vi "Create Configuration From File.vi"(8 "error in (no error)":errorcluster, 10 "Path in":path, 11 "Device Item Ref in":T1 format="%.0x") -> (0 "error out":errorcluster, 3 "Ref out":T1 format="%.0x")   [LabVIEW 2015, in "Diagnostics Addon System Explorer.lvlib"]
uses:
  Diagnostics Addon System Explorer.lvlib
  <vilib>/NI Veristand/Custom Device API/Custom Device Item Ref.ctl
  Types/Exported Configuration.ctl
  Shared/Types/CAN Configuration.ctl
  Shared/Types/CAN Interface.ctl
  Shared/Types/Diagnostic Protocols.ctl
  Shared/Types/Transport Protocols.ctl
  Shared/Types/Security.ctl
  Types/Exported Frames Cluster.ctl
  Shared/Types/Frame Parameters.ctl
  Shared/Types/MessageType Selector.ctl
  Shared/Types/Signal Parameters.ctl
  Types/Exported DPIDs Cluster.ctl
  Types/Exported DPID Parameters.ctl
  Shared/Types/DPID Parameters.ctl
  Shared/Types/DPID Periodic Rate.ctl
  Types/Exported DTC Cluster.ctl
  Shared/Types/Exported DTC Control Cluster.ctl
  Types/Exported 986x Support.ctl
  Types/Exported Command Cluster.ctl
  Types/Exported Status Cluster.ctl
  Shared/Types/Exported IO Control Cluster.ctl
  Shared/Types/IO Control Parameters.ctl
  Shared/Types/Command Response Signals.ctl
  Shared/Types/Exported Routines Cluster.ctl
  Shared/Types/Routine Paramaters.ctl
  <vilib>/NI/GXML/_subVIs/GXML SearchParser/Search Parser.vi
  <vilib>/NI/GXML/GXML.lvlib
  Shared/Diagnostics Addon Shared.lvlib
  <vilib>/NI Veristand/Custom Device API/Custom Device API.lvlib
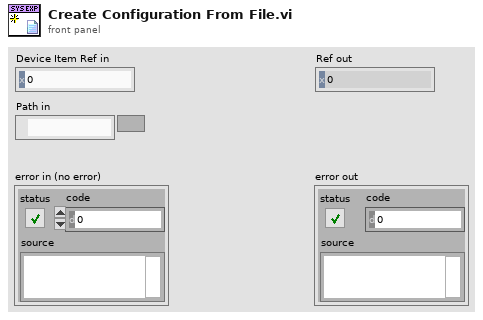
[diagram p1: front panel]
types:
  T1 = typedef "Custom Device API.lvlib/Custom Device Item Ref.ctl" = u64
  T2 = cluster{"Name":string, "Description":string, "Diagnostics Basic Configuraiton":cluster{"Database File":path, "CAN Interface":enum16{"CAN0", "CAN1", "CAN2", "CAN3", "CAN4", "CAN5", "CAN6", "CAN7", "CAN8", "CAN9", "CAN10", "CAN11", "CAN12", "CAN13", "CAN14", "CAN15", "CAN16", "CAN17", "CAN18", "CAN19", "CAN20", "CAN21", "CAN22", "CAN23", "CAN24", "CAN25", "CAN26", "CAN27", "CAN28", "CAN29", "CAN30", "CAN31", "CAN32", "CAN33", "CAN34", "CAN35", "CAN36", "CAN37", "CAN38", "CAN39", "CAN40", "CAN41", "CAN42", "CAN43", "CAN44", "CAN45", "CAN46", "CAN47", "CAN48", "CAN49", "CAN50", "CAN51", "CAN52", "CAN53", "CAN54", "CAN55", "CAN56", "CAN57", "CAN58", "CAN59", "CAN60", "CAN61", "CAN62", "CAN63", "CAN 256 (Virtual)", "CAN 257 (Virtual)"}, "Baud Rate":u32, "Diagnostic Protocol":enum16{"GMLAN", "KWP-2000", "UDS"}, "Transport Protocol":enum16{"ISO TP - Normal Mode", "ISO TP - Mixed Mode", "VW TP 2.0", "Diagnostics on IP"}, "Transmit ID":u32, "Receive ID":u32, "Transmit Extension":u8, "Receive Extension":u8, "Receive UUDT ID":u32, "Enable Stream":bool, "VW TP Channel ID":u32}, "DIDs":cluster{"Description":string, "DIDPID Array":cluster{"Name":string, "Description":string, "ID":u16, "Signals":cluster{"Name":string, "Start Bit":u8, "Length":u8, "Scaling Factor":dbl, "Scaling Offset":dbl, "Minimum":dbl, "Maximum":dbl, "Data Type":u32, "Byte Order":u32, "Default Value":dbl, "Units":string, "Description":string}[]}[]}, "Input PIDs":cluster{"Description":string, "DIDPID Array":cluster{"Name":string, "Description":string, "ID":u16, "Signals":cluster{"Name":string, "Start Bit":u8, "Length":u8, "Scaling Factor":dbl, "Scaling Offset":dbl, "Minimum":dbl, "Maximum":dbl, "Data Type":u32, "Byte Order":u32, "Default Value":dbl, "Units":string, "Description":string}[]}[]}, "Output PIDs":cluster{"Description":string, "DIDPID Array":cluster{"Name":string, "Description":string, "ID":u16, "Signals":cluster{"Name":string, "Start Bit":u8, "Length":u8, "Scaling Factor":dbl, "Scaling Offset":dbl, "Minimum":dbl, "Maximum":dbl, "Data Type":u32, "Byte Order":u32, "Default Value":dbl, "Units":string, "Description":string}[]}[]}, "DPIDs":cluster{"Description":string, "DPIDs":cluster{"Name":string, "Description":string, "DPID":cluster{"DPID ID":u8, "Speed":enum16{"Slow", "Medium", "Fast"}, "PIDs":u16[]}}[]}, "DTC":cluster{"Description":string, "DTC descriptor":cluster{"DTC Byte Length":i32, "Status Byte Length":i32, "Add Data Byte Length":i32, "Byte Order":enum16{"Motorola", "Intel"}}}, "NI 986x Support":cluster{"Enable 986x":bool, "RIO Device":u16, "Bitfile":path}, "Commands":cluster{"Description":string}, "Status":cluster{"Description":string}}
  T3 = typedef "Diagnostics Addon System Explorer.lvlib/Exported Configuration.ctl" = cluster{"Name":string, "Description":string, "Diagnostics Basic Configuraiton":T4, "DIDs":T9, "Input PIDs":T9, "Output PIDs":T9, "DPIDs":T13, "DTC":T17, "NI 986x Support":T19, "Commands":T20, "Status":T21, "IO Controls":T22, "Routines":T25, "Output Memory":T9, "Input Memory":T9}
  T4 = typedef "Diagnostics Addon Shared.lvlib/CAN Configuration.ctl" = cluster{"Database File":path, "CAN Interface":T5, "Baud Rate":u32, "Diagnostic Protocol":T6, "Transport Protocol":T7, "Transmit ID":u32, "Receive ID":u32, "Transmit Extension":u8, "Receive Extension":u8, "Receive UUDT ID":u32, "Enable Stream":bool, "VW TP Channel ID":u32, "Security":T8, "Fill Frame":bool, "Fill Byte":u8, "Termination":bool}
  T5 = typedef "Diagnostics Addon Shared.lvlib/CAN Interface.ctl" = enum16{"CAN0", "CAN1", "CAN2", "CAN3", "CAN4", "CAN5", "CAN6", "CAN7", "CAN8", "CAN9", "CAN10", "CAN11", "CAN12", "CAN13", "CAN14", "CAN15", "CAN16", "CAN17", "CAN18", "CAN19", "CAN20", "CAN21", "CAN22", "CAN23", "CAN24", "CAN25", "CAN26", "CAN27", "CAN28", "CAN29", "CAN30", "CAN31", "CAN32", "CAN33", "CAN34", "CAN35", "CAN36", "CAN37", "CAN38", "CAN39", "CAN40", "CAN41", "CAN42", "CAN43", "CAN44", "CAN45", "CAN46", "CAN47", "CAN48", "CAN49", "CAN50", "CAN51", "CAN52", "CAN53", "CAN54", "CAN55", "CAN56", "CAN57", "CAN58", "CAN59", "CAN60", "CAN61", "CAN62", "CAN63", "CAN 256 (Virtual)", "CAN 257 (Virtual)"}
  T6 = typedef "Diagnostics Addon Shared.lvlib/Diagnostic Protocols.ctl" = enum16{"GMLAN", "KWP-2000", "UDS"}
  T7 = typedef "Diagnostics Addon Shared.lvlib/Transport Protocols.ctl" = enum16{"ISO TP - Normal Mode", "ISO TP - Mixed Mode", "VW TP 2.0", "Diagnostics on IP"}
  T8 = typedef "Diagnostics Addon Shared.lvlib/Security.ctl" = cluster{"Source DLL Path":path, "Security Level":u8, "Target DLL Path":path}
  T9 = typedef "Diagnostics Addon System Explorer.lvlib/Exported Frames Cluster.ctl" = cluster{"Description":string, "Frames":T10[]}
  T10 = typedef "Diagnostics Addon Shared.lvlib/Frame Parameters.ctl" = cluster{"Name":string, "Description":string, "ID":u32, "Type":T11, "Signals":T12[]}
  T11 = typedef "Diagnostics Addon Shared.lvlib/MessageType Selector.ctl" = enum16{"DID", "PID", "CPID", "Write Memory", "Read Memory", "DTC Control", "IO Cmd", "IO Resp", "Routine Start Cmd", "Routine Start Resp", "Routine Status Cmd", "Routine Status Resp", "Routine Stop Cmd", "Routine Stop Resp"}
  T12 = typedef "Diagnostics Addon Shared.lvlib/Signal Parameters.ctl" = cluster{"Start Bit":u8, "Length":u8, "Scaling Factor":dbl, "Scaling Offset":dbl, "Minimum":dbl, "Maximum":dbl, "Data Type":u32, "Byte Order":u32, "Default Value":dbl, "Name":string, "Units":string, "Description":string}
  T13 = typedef "Diagnostics Addon System Explorer.lvlib/Exported DPIDs Cluster.ctl" = cluster{"Description":string, "DPIDs":T14[]}
  T14 = typedef "Diagnostics Addon System Explorer.lvlib/Exported DPID Parameters.ctl" = cluster{"Name":string, "Description":string, "DPID":T15}
  T15 = typedef "Diagnostics Addon Shared.lvlib/DPID Parameters.ctl" = cluster{"DPID ID":u8, "Speed":T16, "PIDs":u16[]}
  T16 = typedef "Diagnostics Addon Shared.lvlib/DPID Periodic Rate.ctl" = enum16{"Slow", "Medium", "Fast"}
  T17 = typedef "Diagnostics Addon System Explorer.lvlib/Exported DTC Cluster.ctl" = cluster{"Description":string, "DTC descriptor":cluster{"DTC Byte Length":i32, "Status Byte Length":i32, "Add Data Byte Length":i32, "Byte Order":enum16{"Motorola", "Intel"}}, "DTCControl":T18}
  T18 = typedef "Diagnostics Addon Shared.lvlib/Exported DTC Control Cluster.ctl" = cluster{"Description":string, "Signals":T12[]}
  T19 = typedef "Diagnostics Addon System Explorer.lvlib/Exported 986x Support.ctl" = cluster{"Enable 986x":bool, "RIO Device":u16, "Bitfile":path}
  T20 = typedef "Diagnostics Addon System Explorer.lvlib/Exported Command Cluster.ctl" = cluster{"Description":string}
  T21 = typedef "Diagnostics Addon System Explorer.lvlib/Exported Status Cluster.ctl" = cluster{"Description":string}
  T22 = typedef "Diagnostics Addon Shared.lvlib/Exported IO Control Cluster.ctl" = cluster{"Description":string, "IO Control Array":T23[]}
  T23 = typedef "Diagnostics Addon Shared.lvlib/IO Control Parameters.ctl" = cluster{"Name":string, "Description":string, "ID":u16, "Signals":T24}
  T24 = typedef "Diagnostics Addon Shared.lvlib/Command Response Signals.ctl" = cluster{"Cmd":T12[], "Response":T12[]}
  T25 = typedef "Diagnostics Addon Shared.lvlib/Exported Routines Cluster.ctl" = cluster{"Description":string, "Routine Array":T26[]}
  T26 = typedef "Diagnostics Addon Shared.lvlib/Routine Paramaters.ctl" = cluster{"Name":string, "Description":string, "ID":u16, "Start Parameters":T24, "Request Parameters":T24, "Stop Parameters":T24}
  T27 = cluster{"Description":string, "DPIDs":cluster{"Name":string, "Description":string, "DPID":cluster{"DPID ID":u8, "Speed":enum16{"Slow", "Medium", "Fast"}, "PIDs":u16[]}}[]}
  T28 = cluster{"DTC Byte Length":i32, "Status Byte Length":i32, "Add Data Byte Length":i32, "Byte Order":enum16{"Motorola", "Intel"}}
  T29 = cluster{"Enable 986x":bool, "RIO Device":u16, "Bitfile":path}
  T30 = enum16{"CAN0", "CAN1", "CAN2", "CAN3", "CAN4", "CAN5", "CAN6", "CAN7", "CAN8", "CAN9", "CAN10", "CAN11", "CAN12", "CAN13", "CAN14", "CAN15", "CAN16", "CAN17", "CAN18", "CAN19", "CAN20", "CAN21", "CAN22", "CAN23", "CAN24", "CAN25", "CAN26", "CAN27", "CAN28", "CAN29", "CAN30", "CAN31", "CAN32", "CAN33", "CAN34", "CAN35", "CAN36", "CAN37", "CAN38", "CAN39", "CAN40", "CAN41", "CAN42", "CAN43", "CAN44", "CAN45", "CAN46", "CAN47", "CAN48", "CAN49", "CAN50", "CAN51", "CAN52", "CAN53", "CAN54", "CAN55", "CAN56", "CAN57", "CAN58", "CAN59", "CAN60", "CAN61", "CAN62", "CAN63", "CAN 256 (Virtual)", "CAN 257 (Virtual)"}
  T31 = enum16{"ISO TP - Normal Mode", "ISO TP - Mixed Mode", "VW TP 2.0", "Diagnostics on IP"}
  T32 = cluster{"Name":string, "Description":string, "ID":u16, "Signals":cluster{"Name":string, "Start Bit":u8, "Length":u8, "Scaling Factor":dbl, "Scaling Offset":dbl, "Minimum":dbl, "Maximum":dbl, "Data Type":u32, "Byte Order":u32, "Default Value":dbl, "Units":string, "Description":string}[]}[]
  T33 = cluster{"Name":string, "Description":string, "Diagnostics Basic Configuraiton":cluster{"Database File":path, "CAN Interface":enum16{"CAN0", "CAN1", "CAN2", "CAN3", "CAN4", "CAN5", "CAN6", "CAN7", "CAN8", "CAN9", "CAN10", "CAN11", "CAN12", "CAN13", "CAN14", "CAN15", "CAN16", "CAN17", "CAN18", "CAN19", "CAN20", "CAN21", "CAN22", "CAN23", "CAN24", "CAN25", "CAN26", "CAN27", "CAN28", "CAN29", "CAN30", "CAN31", "CAN32", "CAN33", "CAN34", "CAN35", "CAN36", "CAN37", "CAN38", "CAN39", "CAN40", "CAN41", "CAN42", "CAN43", "CAN44", "CAN45", "CAN46", "CAN47", "CAN48", "CAN49", "CAN50", "CAN51", "CAN52", "CAN53", "CAN54", "CAN55", "CAN56", "CAN57", "CAN58", "CAN59", "CAN60", "CAN61", "CAN62", "CAN63", "CAN 256 (Virtual)", "CAN 257 (Virtual)"}, "Baud Rate":u32, "Diagnostic Protocol":enum16{"GMLAN", "KWP-2000", "UDS"}, "Transport Protocol":enum16{"ISO TP - Normal Mode", "ISO TP - Mixed Mode", "VW TP 2.0", "Diagnostics on IP"}, "Transmit ID":u32, "Receive ID":u32, "Transmit Extension":u8, "Receive Extension":u8, "Receive UUDT ID":u32, "Enable Stream":bool, "VW TP Channel ID":u32}, "DIDs":cluster{"Description":string, "DIDPID Array":cluster{"Name":string, "Description":string, "ID":u16, "Signals":cluster{"Start Bit":u8, "Length":u8, "Scaling Factor":dbl, "Scaling Offset":dbl, "Minimum":dbl, "Maximum":dbl, "Data Type":u32, "Byte Order":u32, "Default Value":dbl, "Name":string, "Units":string, "Description":string}[]}[]}, "Input PIDs":cluster{"Description":string, "DIDPID Array":cluster{"Name":string, "Description":string, "ID":u16, "Signals":cluster{"Start Bit":u8, "Length":u8, "Scaling Factor":dbl, "Scaling Offset":dbl, "Minimum":dbl, "Maximum":dbl, "Data Type":u32, "Byte Order":u32, "Default Value":dbl, "Name":string, "Units":string, "Description":string}[]}[]}, "Output PIDs":cluster{"Description":string, "DIDPID Array":cluster{"Name":string, "Description":string, "ID":u16, "Signals":cluster{"Start Bit":u8, "Length":u8, "Scaling Factor":dbl, "Scaling Offset":dbl, "Minimum":dbl, "Maximum":dbl, "Data Type":u32, "Byte Order":u32, "Default Value":dbl, "Name":string, "Units":string, "Description":string}[]}[]}, "DPIDs":cluster{"Description":string, "DPIDs":cluster{"Name":string, "Description":string, "DPID":cluster{"DPID ID":u8, "Speed":enum16{"Slow", "Medium", "Fast"}, "PIDs":u16[]}}[]}, "DTC":cluster{"Description":string, "DTC descriptor":cluster{"DTC Byte Length":i32, "Status Byte Length":i32, "Add Data Byte Length":i32, "Byte Order":enum16{"Motorola", "Intel"}}}, "NI 986x Support":cluster{"Enable 986x":bool, "RIO Device":u16, "Bitfile":path}, "Commands":cluster{"Description":string}, "Status":cluster{"Description":string}}
  T34 = cluster{"Name":string, "Description":string, "ID":u16, "Signals":cluster{"Start Bit":u8, "Length":u8, "Scaling Factor":dbl, "Scaling Offset":dbl, "Minimum":dbl, "Maximum":dbl, "Data Type":u32, "Byte Order":u32, "Default Value":dbl, "Name":string, "Units":string, "Description":string}[]}[]
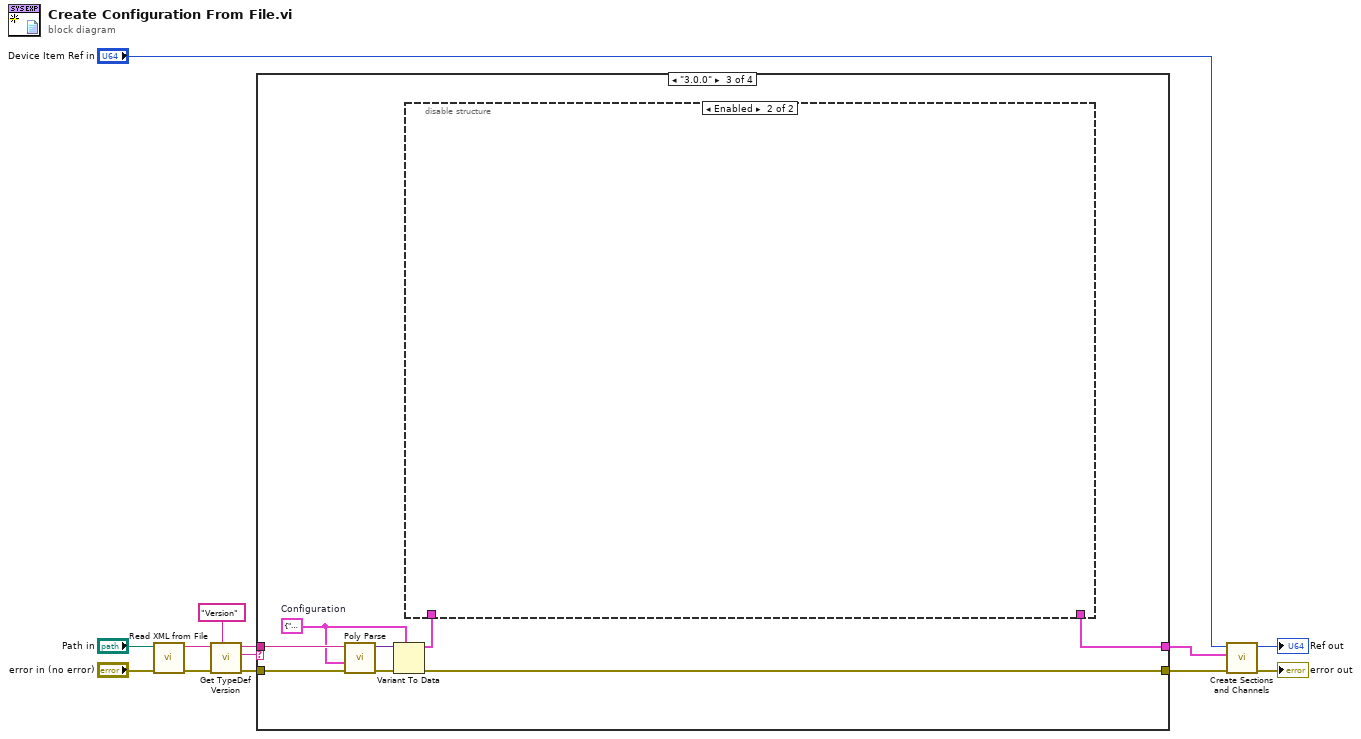
[diagram p0: block diagram]
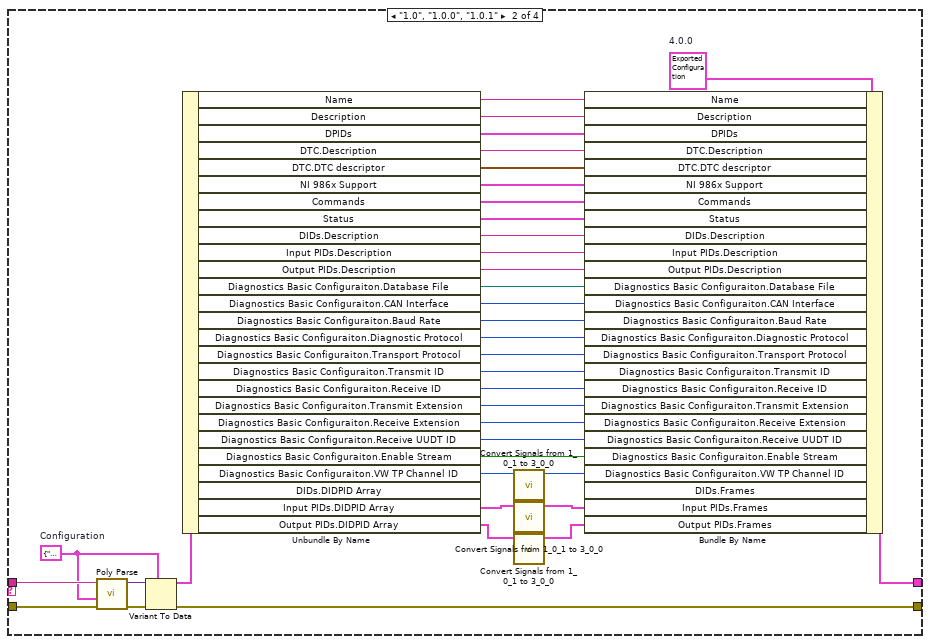
[diagram p3: hidden frame]
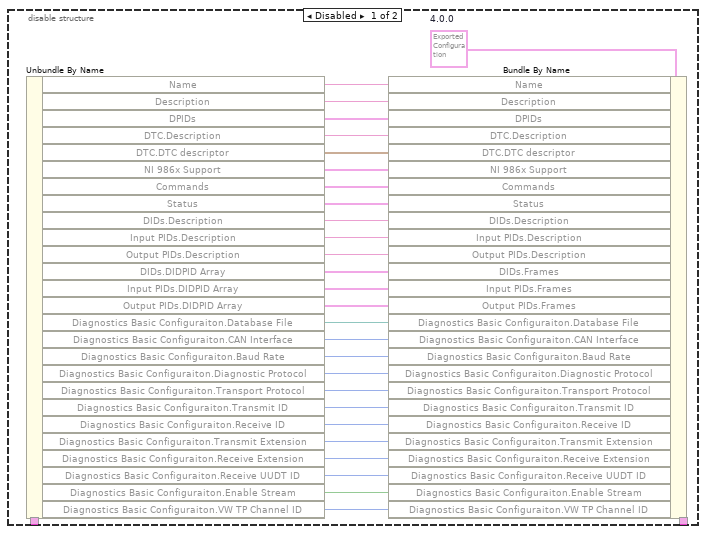
[diagram p4: hidden frame]
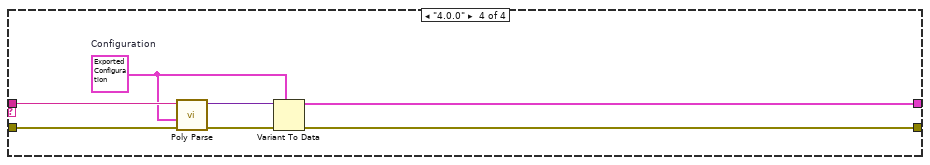
[diagram p5: hidden frame]
diagram:
  n1 = call <vilib>:"Read XML from File.vi"("error in"="error in (no error)", "XML File Path"="Path in") -> ("error out"=w13:errorcluster, "XML String Out"=w12:string)  [unwired: 8 in]
  n2 = call <vilib>:"Get TypeDef Version.vi"("Version Tag Name"="Version", "error in"=w13, "XML String In"=w12) -> ("error out"=w9:errorcluster, "Version String"=w8:string, "XML String Out"=w10:string)  [unwired: 6 in]
  n3 = case shown="\"3.0.0\"" w8 {
    tunnel: w10 -> [_ w52 w60 w96]
    tunnel: w9 -> [w14 w51 w59 w95]
    tunnel: [_ w35 w54 w92] -> w1
    tunnel: [w14 w48 w56 w90] -> w5
    frame Default {
    }
    frame "1.0", "1.0.0", "1.0.1" {
      w34 = T2 {"Name"="", "Description"="", "Diagnostics Basic Configuraiton"={"Database File"=path "", "CAN Interface"=enum."CAN0", "Baud Rate"=0, "Diagnostic Protocol"=enum."GMLAN", "Transport Protocol"=enum."ISO TP - Normal Mode", "Transmit ID"=0, "Receive ID"=0, "Transmit Extension"=0, "Receive Extension"=0, "Receive UUDT ID"=0, "Enable Stream"=FALSE, "VW TP Channel ID"=0}, "DIDs"={"Description"="", "DIDPID Array"=[]}, "Input PIDs"={"Description"="", "DIDPID Array"=[]}, "Output PIDs"={"Description"="", "DIDPID Array"=[]}, "DPIDs"={"Description"="", "DPIDs"=[]}, "DTC"={"Description"="", "DTC descriptor"={"DTC Byte Length"=0, "Status Byte Length"=0, "Add Data Byte Length"=0, "Byte Order"=enum."Motorola"}}, "NI 986x Support"={"Enable 986x"=FALSE, "RIO Device"=0, "Bitfile"=path ""}, "Commands"={"Description"=""}, "Status"={"Description"=""}}  # Configuration
      w46 = T3 {"Name"="", "Description"="", "Diagnostics Basic Configuraiton"={"Database File"=path "", "CAN Interface"=enum."CAN0", "Baud Rate"=0, "Diagnostic Protocol"=enum."GMLAN", "Transport Protocol"=enum."ISO TP - Normal Mode", "Transmit ID"=0, "Receive ID"=0, "Transmit Extension"=0, "Receive Extension"=0, "Receive UUDT ID"=0, "Enable Stream"=FALSE, "VW TP Channel ID"=0, "Security"={"Source DLL Path"=path "", "Security Level"=1, "Target DLL Path"=path ""}, "Fill Frame"=FALSE, "Fill Byte"=255, "Termination"=FALSE}, "DIDs"={"Description"="", "Frames"=[]}, "Input PIDs"={"Description"="", "Frames"=[]}, "Output PIDs"={"Description"="", "Frames"=[]}, "DPIDs"={"Description"="", "DPIDs"=[]}, "DTC"={"Description"="", "DTC descriptor"={"DTC Byte Length"=0, "Status Byte Length"=0, "Add Data Byte Length"=0, "Byte Order"=enum."Motorola"}, "DTCControl"={"Description"="", "Signals"=[]}}, "NI 986x Support"={"Enable 986x"=FALSE, "RIO Device"=0, "Bitfile"=path ""}, "Commands"={"Description"=""}, "Status"={"Description"=""}, "IO Controls"={"Description"="", "IO Control Array"=[]}, "Routines"={"Description"="", "Routine Array"=[]}, "Output Memory"={"Description"="", "Frames"=[]}, "Input Memory"={"Description"="", "Frames"=[]}}  # 4.0.0
      n4 = call-poly <vilib>:"Poly Parse.vi"("error in"=w51, "TypeDesc"=w34, "XML String In"=w52) -> ("error out"=w50:errorcluster, "Parsed Data"=w49:variant)  [unwired: 7 in]
      n5 = Variant To Data(error in=w50, type=w34, Variant=w49) -> (data=w47:T2, error out=w48:errorcluster)
      n6 = Unbundle By Name(w47) -> ("Name"=w45:string, "Description"=w44:string, "DPIDs"=w43:T27, "DTC.Description"=w39:string, "DTC.DTC descriptor"=w15:T28, "NI 986x Support"=w40:T29, "Commands"=w41:cluster{"Description":string}, "Status"=w42:cluster{"Description":string}, "DIDs.Description"=w38:string, "Input PIDs.Description"=w37:string, "Output PIDs.Description"=w36:string, "Diagnostics Basic Configuraiton.Database File"=w22:path, "Diagnostics Basic Configuraiton.CAN Interface"=w23:T30, "Diagnostics Basic Configuraiton.Baud Rate"=w24:u32, "Diagnostics Basic Configuraiton.Diagnostic Protocol"=w25:enum16{"GMLAN", "KWP-2000", "UDS"}, "Diagnostics Basic Configuraiton.Transport Protocol"=w26:T31, "Diagnostics Basic Configuraiton.Transmit ID"=w27:u32, "Diagnostics Basic Configuraiton.Receive ID"=w28:u32, "Diagnostics Basic Configuraiton.Transmit Extension"=w29:u8, "Diagnostics Basic Configuraiton.Receive Extension"=w30:u8, "Diagnostics Basic Configuraiton.Receive UUDT ID"=w31:u32, "Diagnostics Basic Configuraiton.Enable Stream"=w32:bool, "Diagnostics Basic Configuraiton.VW TP Channel ID"=w33:u32, "DIDs.DIDPID Array"=w21:T32, "Input PIDs.DIDPID Array"=w20:T32, "Output PIDs.DIDPID Array"=w19:T32)
      n7 = call "Convert Signals from 1_0_1 to 3_0_0.vi"("Signals"=w21) -> ("Signals"=w18:T10[])  [unwired: 10 in]
      n8 = call "Convert Signals from 1_0_1 to 3_0_0.vi"("Signals"=w20) -> ("Signals"=w17:T10[])  [unwired: 10 in]
      n9 = call "Convert Signals from 1_0_1 to 3_0_0.vi"("Signals"=w19) -> ("Signals"=w16:T10[])  [unwired: 10 in]
      n10 = Bundle By Name(cluster=w46, "Name"=w45, "Description"=w44, "DPIDs"=w43, "DTC.Description"=w39, "DTC.DTC descriptor"=w15, "NI 986x Support"=w40, "Commands"=w41, "Status"=w42, "DIDs.Description"=w38, "Input PIDs.Description"=w37, "Output PIDs.Description"=w36, "Diagnostics Basic Configuraiton.Database File"=w22, "Diagnostics Basic Configuraiton.CAN Interface"=w23, "Diagnostics Basic Configuraiton.Baud Rate"=w24, "Diagnostics Basic Configuraiton.Diagnostic Protocol"=w25, "Diagnostics Basic Configuraiton.Transport Protocol"=w26, "Diagnostics Basic Configuraiton.Transmit ID"=w27, "Diagnostics Basic Configuraiton.Receive ID"=w28, "Diagnostics Basic Configuraiton.Transmit Extension"=w29, "Diagnostics Basic Configuraiton.Receive Extension"=w30, "Diagnostics Basic Configuraiton.Receive UUDT ID"=w31, "Diagnostics Basic Configuraiton.Enable Stream"=w32, "Diagnostics Basic Configuraiton.VW TP Channel ID"=w33, "DIDs.Frames"=w18, "Input PIDs.Frames"=w17, "Output PIDs.Frames"=w16) -> (w35:T3)
    }
    frame "3.0.0" {
      w53 = T33 {"Name"="", "Description"="", "Diagnostics Basic Configuraiton"={"Database File"=path "", "CAN Interface"=enum."CAN0", "Baud Rate"=0, "Diagnostic Protocol"=enum."GMLAN", "Transport Protocol"=enum."ISO TP - Normal Mode", "Transmit ID"=0, "Receive ID"=0, "Transmit Extension"=0, "Receive Extension"=0, "Receive UUDT ID"=0, "Enable Stream"=FALSE, "VW TP Channel ID"=0}, "DIDs"={"Description"="", "DIDPID Array"=[]}, "Input PIDs"={"Description"="", "DIDPID Array"=[]}, "Output PIDs"={"Description"="", "DIDPID Array"=[]}, "DPIDs"={"Description"="", "DPIDs"=[]}, "DTC"={"Description"="", "DTC descriptor"={"DTC Byte Length"=0, "Status Byte Length"=0, "Add Data Byte Length"=0, "Byte Order"=enum."Motorola"}}, "NI 986x Support"={"Enable 986x"=FALSE, "RIO Device"=0, "Bitfile"=path ""}, "Commands"={"Description"=""}, "Status"={"Description"=""}}  # Configuration
      n11 = call-poly <vilib>:"Poly Parse.vi"("error in"=w59, "TypeDesc"=w53, "XML String In"=w60) -> ("error out"=w58:errorcluster, "Parsed Data"=w57:variant)  [unwired: 7 in]
      n12 = Variant To Data(error in=w58, type=w53, Variant=w57) -> (data=w55:T33, error out=w56:errorcluster)
      n13 = disable-structure shown="Enabled" {
        disable-tunnel: w55 -> [w89 _]
        disable-tunnel: [w77 _] -> w54
        frame Disabled {
          w88 = T3 {"Name"="", "Description"="", "Diagnostics Basic Configuraiton"={"Database File"=path "", "CAN Interface"=enum."CAN0", "Baud Rate"=0, "Diagnostic Protocol"=enum."GMLAN", "Transport Protocol"=enum."ISO TP - Normal Mode", "Transmit ID"=0, "Receive ID"=0, "Transmit Extension"=0, "Receive Extension"=0, "Receive UUDT ID"=0, "Enable Stream"=FALSE, "VW TP Channel ID"=0, "Security"={"Source DLL Path"=path "", "Security Level"=1, "Target DLL Path"=path ""}, "Fill Frame"=FALSE, "Fill Byte"=255, "Termination"=FALSE}, "DIDs"={"Description"="", "Frames"=[]}, "Input PIDs"={"Description"="", "Frames"=[]}, "Output PIDs"={"Description"="", "Frames"=[]}, "DPIDs"={"Description"="", "DPIDs"=[]}, "DTC"={"Description"="", "DTC descriptor"={"DTC Byte Length"=0, "Status Byte Length"=0, "Add Data Byte Length"=0, "Byte Order"=enum."Motorola"}, "DTCControl"={"Description"="", "Signals"=[]}}, "NI 986x Support"={"Enable 986x"=FALSE, "RIO Device"=0, "Bitfile"=path ""}, "Commands"={"Description"=""}, "Status"={"Description"=""}, "IO Controls"={"Description"="", "IO Control Array"=[]}, "Routines"={"Description"="", "Routine Array"=[]}, "Output Memory"={"Description"="", "Frames"=[]}, "Input Memory"={"Description"="", "Frames"=[]}}  # 4.0.0
          n14 = Unbundle By Name(w89) -> ("Name"=w87:string, "Description"=w86:string, "DPIDs"=w85:T27, "DTC.Description"=w81:string, "DTC.DTC descriptor"=w61:T28, "NI 986x Support"=w82:T29, "Commands"=w83:cluster{"Description":string}, "Status"=w84:cluster{"Description":string}, "DIDs.Description"=w80:string, "Input PIDs.Description"=w79:string, "Output PIDs.Description"=w78:string, "DIDs.DIDPID Array"=w76:T34, "Input PIDs.DIDPID Array"=w75:T34, "Output PIDs.DIDPID Array"=w74:T34, "Diagnostics Basic Configuraiton.Database File"=w62:path, "Diagnostics Basic Configuraiton.CAN Interface"=w63:T30, "Diagnostics Basic Configuraiton.Baud Rate"=w64:u32, "Diagnostics Basic Configuraiton.Diagnostic Protocol"=w65:enum16{"GMLAN", "KWP-2000", "UDS"}, "Diagnostics Basic Configuraiton.Transport Protocol"=w66:T31, "Diagnostics Basic Configuraiton.Transmit ID"=w67:u32, "Diagnostics Basic Configuraiton.Receive ID"=w68:u32, "Diagnostics Basic Configuraiton.Transmit Extension"=w69:u8, "Diagnostics Basic Configuraiton.Receive Extension"=w70:u8, "Diagnostics Basic Configuraiton.Receive UUDT ID"=w71:u32, "Diagnostics Basic Configuraiton.Enable Stream"=w72:bool, "Diagnostics Basic Configuraiton.VW TP Channel ID"=w73:u32)
          n15 = Bundle By Name(cluster=w88, "Name"=w87, "Description"=w86, "DPIDs"=w85, "DTC.Description"=w81, "DTC.DTC descriptor"=w61, "NI 986x Support"=w82, "Commands"=w83, "Status"=w84, "DIDs.Description"=w80, "Input PIDs.Description"=w79, "Output PIDs.Description"=w78, "DIDs.Frames"=w76, "Input PIDs.Frames"=w75, "Output PIDs.Frames"=w74, "Diagnostics Basic Configuraiton.Database File"=w62, "Diagnostics Basic Configuraiton.CAN Interface"=w63, "Diagnostics Basic Configuraiton.Baud Rate"=w64, "Diagnostics Basic Configuraiton.Diagnostic Protocol"=w65, "Diagnostics Basic Configuraiton.Transport Protocol"=w66, "Diagnostics Basic Configuraiton.Transmit ID"=w67, "Diagnostics Basic Configuraiton.Receive ID"=w68, "Diagnostics Basic Configuraiton.Transmit Extension"=w69, "Diagnostics Basic Configuraiton.Receive Extension"=w70, "Diagnostics Basic Configuraiton.Receive UUDT ID"=w71, "Diagnostics Basic Configuraiton.Enable Stream"=w72, "Diagnostics Basic Configuraiton.VW TP Channel ID"=w73) -> (w77:T3)
        }
        frame Enabled {
        }
      }
    }
    frame "4.0.0" {
      w91 = T3 {"Name"="", "Description"="", "Diagnostics Basic Configuraiton"={"Database File"=path "", "CAN Interface"=enum."CAN0", "Baud Rate"=0, "Diagnostic Protocol"=enum."GMLAN", "Transport Protocol"=enum."ISO TP - Normal Mode", "Transmit ID"=0, "Receive ID"=0, "Transmit Extension"=0, "Receive Extension"=0, "Receive UUDT ID"=0, "Enable Stream"=FALSE, "VW TP Channel ID"=0, "Security"={"Source DLL Path"=path "", "Security Level"=1, "Target DLL Path"=path ""}, "Fill Frame"=FALSE, "Fill Byte"=255, "Termination"=FALSE}, "DIDs"={"Description"="", "Frames"=[]}, "Input PIDs"={"Description"="", "Frames"=[]}, "Output PIDs"={"Description"="", "Frames"=[]}, "DPIDs"={"Description"="", "DPIDs"=[]}, "DTC"={"Description"="", "DTC descriptor"={"DTC Byte Length"=0, "Status Byte Length"=0, "Add Data Byte Length"=0, "Byte Order"=enum."Motorola"}, "DTCControl"={"Description"="", "Signals"=[]}}, "NI 986x Support"={"Enable 986x"=FALSE, "RIO Device"=0, "Bitfile"=path ""}, "Commands"={"Description"=""}, "Status"={"Description"=""}, "IO Controls"={"Description"="", "IO Control Array"=[]}, "Routines"={"Description"="", "Routine Array"=[]}, "Output Memory"={"Description"="", "Frames"=[]}, "Input Memory"={"Description"="", "Frames"=[]}}  # Configuration
      n16 = call-poly <vilib>:"Poly Parse.vi"("error in"=w95, "TypeDesc"=w91, "XML String In"=w96) -> ("error out"=w94:errorcluster, "Parsed Data"=w93:variant)  [unwired: 7 in]
      n17 = Variant To Data(error in=w94, type=w91, Variant=w93) -> (data=w92:T3, error out=w90:errorcluster)
    }
  }
  n18 = call "Create Sections and Channels.vi"("error in (no error)"=w5, "Configuration"=w1, "Device Item Ref in"="Device Item Ref in") -> ("error out"=→"error out":errorcluster, "Device Item Ref out"=→"Ref out":T1)  [unwired: 7 in]
